vi "test max speed.vi"() -> ()   [LabVIEW 2018]
uses:
  type defs/tet max speed enum.ctl
  <vilib>/Instr/_visa.llb/VISA Configure Serial Port (Instr).vi
panel:
  in  "stop":bool
  out "error IO":errorcluster
  in  "pan tilt stop":bool
  in  "turbo tilt speed":bool
  in  "max tilt speed":bool
  in  "turbo pan speed":bool
  in  "max pan speed":bool
  in  "connect":bool
  in  "VISA resource name":refnum<visa-resource-name>="COM6"
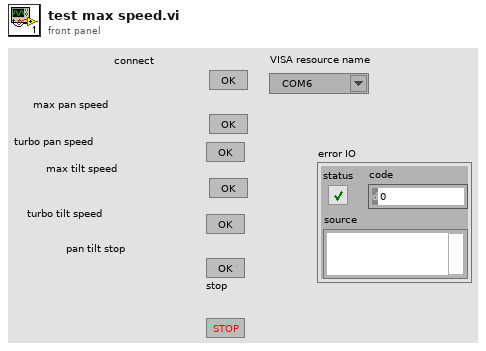
[diagram p1: front panel]
types:
  T1 = typedef "tet max speed enum.ctl" = enum16{"event", "write", "step1", "exit"}
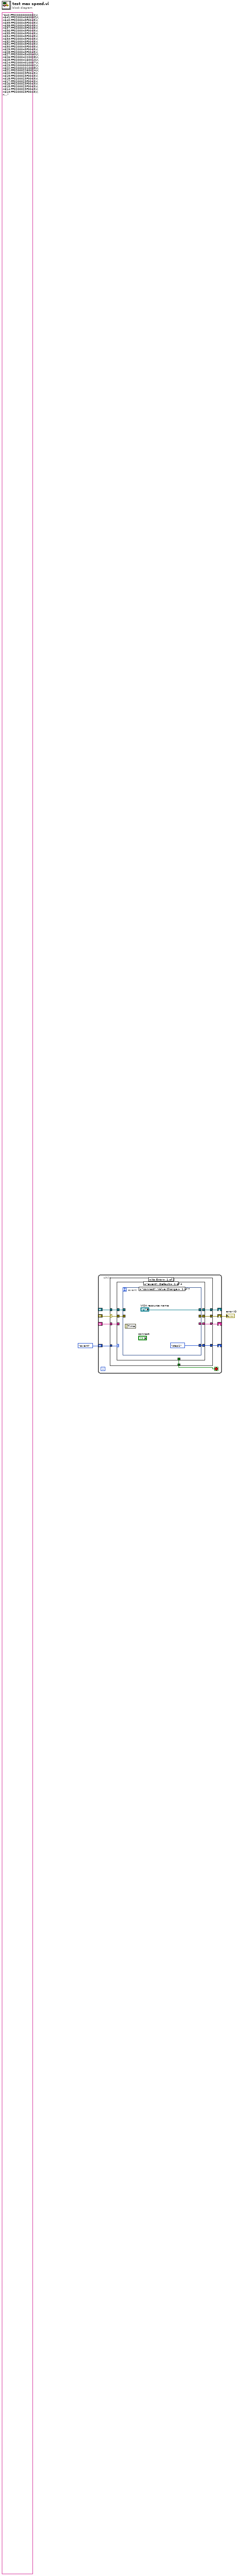
[diagram p0: block diagram]
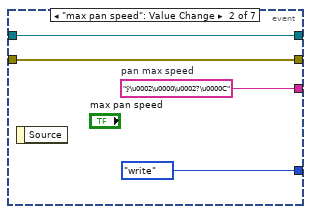
[diagram p2: hidden frame]
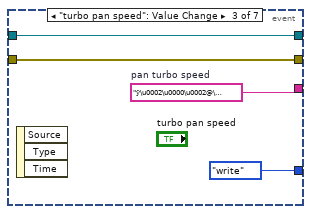
[diagram p3: hidden frame]
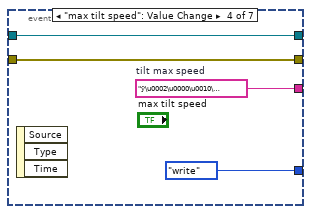
[diagram p4: hidden frame]
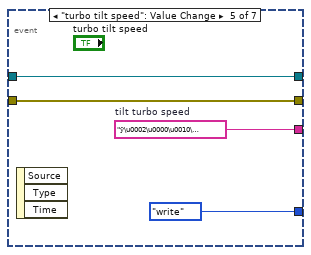
[diagram p5: hidden frame]
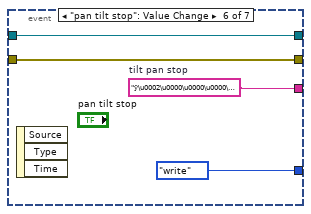
[diagram p6: hidden frame]
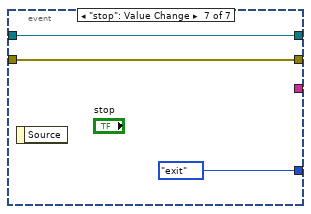
[diagram p7: hidden frame]
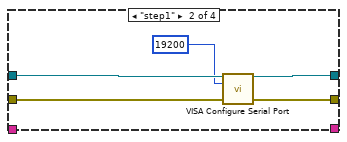
[diagram p8: hidden frame]
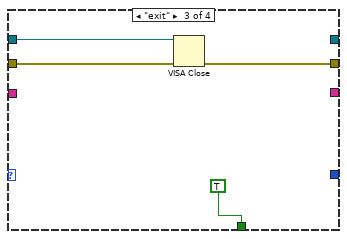
[diagram p9: hidden frame]
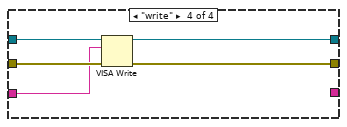
[diagram p10: hidden frame]
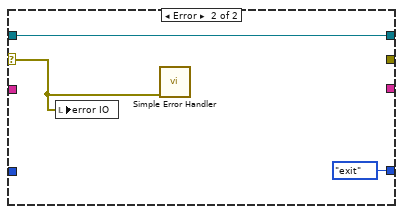
[diagram p11: hidden frame]
diagram:
  (unwired) "642:FF020000000002\r\n641:FF02000406000C\r\n640:FF0200043F0045\r\n639:FF0200043F0045\r\n638:FF0200043F0045\r\n637:FF0200043F0045\r\n636:FF0200043F0045\r\n635:FF0200043F0045\r\n634:FF0200043F0045\r\n633:FF0200043F0045\r\n632:FF0200043F0045\r\n631:FF0200043F0045\r\n630:FF0200043F0045\r\n629:FF0200043F0045\r\n628:FF0200043F0045\r\n627:FF0200043A0040\r\n626:FF020004220028\r\n625:FF02000416001C\r\n624:FF020004010007\r\n623:FF020000000002\r\n622:FF020002010005\r\n621:FF02000226002A\r\n620:FF0200023F0043\r\n619:FF0200023F0043\r\n618:FF0200023F0043\r\n617:FF0200023F0043\r\n616:FF0200023F0043\r\n615:FF0200023F0043\r\n614:FF0200023F0043\r\n613:FF0200023F0043\r\n612:FF0200023F0043\r\n611:FF0200023F0043\r\n610:FF0200023E0042\r\n609:FF02000236003A\r\n608:FF0200021D0021\r\n607:FF020002010005\r\n606:FF0200020E0012\r\n605:FF02000238003C\r\n604:FF0200023F0043\r\n603:FF0200023F0043\r\n602:FF0200023F0043\r\n601:FF0200023F0043\r\n600:FF0200023F0043\r\n599:FF0200023F0043\r\n598:FF0200023F0043\r\n597:FF0200023F0043\r\n596:FF0200023F0043\r\n595:FF02000238003C\r\n594:FF020002240028\r\n593:FF0200021C0020\r\n592:FF020002110015\r\n591:FF020002010005\r\n590:FF0200042A0030\r\n589:FF0200043F0045\r\n588:FF0200043F0045\r\n587:FF0200043F0045\r\n586:FF0200043F0045\r\n585:FF0200043F0045\r\n584:FF0200043F0045\r\n583:FF0200043F0045\r\n582:FF0200043E0044\r\n581:FF0200043F0045\r\n580:FF0200043E0044\r\n579:FF0200043F0045\r\n578:FF0200043F0045\r\n577:FF0200043F0045\r\n576:FF0200043F0045\r\n575:FF0200043F0045\r\n574:FF0200043E0044\r\n573:FF0200043F0045\r\n572:FF0200043F0045\r\n571:FF0200043F0045\r\n570:FF0200043F0045\r\n569:FF0200043F0045\r\n568:FF0200043E0044\r\n567:FF0200043F0045\r\n566:FF0200043F0045\r\n565:FF0200043F0045\r\n564:FF0200043F0045\r\n563:FF0200043E0044\r\n562:FF0200043F0045\r\n561:FF0200043E0044\r\n560:FF020004010007\r\n559:FF020000000002\r\n558:FF020002140018\r\n557:FF0200022E0032\r\n556:FF0200023F0043\r\n555:FF0200023F0043\r\n554:FF0200023F0043\r\n553:FF0200023F0043\r\n552:FF0200023F0043\r\n551:FF0200023F0043\r\n550:FF0200023F0043\r\n549:FF0200023F0043\r\n548:FF0200023F0043\r\n547:FF0200023F0043\r\n546:FF0200023F0043\r\n545:FF0200023F0043\r\n544:FF0200023F0043\r\n543:FF0200023F0043\r\n542:FF0200023F0043\r\n541:FF0200023F0043\r\n540:FF0200023F0043\r\n539:FF0200023F0043\r\n538:FF0200023F0043\r\n537:FF0200023F0043\r\n536:FF0200023F0043\r\n535:FF0200023F0043\r\n534:FF0200023F0043\r\n533:FF0200023F0043\r\n532:FF0200023F0043\r\n531:FF0200023F0043\r\n530:FF0200023F0043\r\n529:FF0200023F0043\r\n528:FF020002340038\r\n527:FF0200022C0030\r\n526:FF020002220026\r\n525:FF020002110015\r\n524:FF020002010005\r\n523:FF0200041E0024\r\n522:FF0200043F0045\r\n521:FF0200043E0044\r\n520:FF0200043F0045\r\n519:FF0200043F0045\r\n518:FF0200043F0045\r\n517:FF0200043F0045\r\n516:FF0200043F0045\r\n515:FF0200043F0045\r\n514:FF0200043F0045\r\n513:FF0200043F0045\r\n512:FF0200043F0045\r\n511:FF0200043E0044\r\n510:FF02000438003E\r\n509:FF02000428002E\r\n508:FF0200040D0013\r\n507:FF020004010007\r\n506:FF020000000002\r\n505:FF02000226002A\r\n504:FF0200023F0043\r\n503:FF0200023F0043\r\n502:FF0200023F0043\r\n501:FF0200023F0043\r\n500:FF0200023F0043\r\n499:FF0200023F0043\r\n498:FF0200023F0043\r\n497:FF0200023F0043\r\n496:FF0200023F0043\r\n495:FF0200023F0043\r\n494:FF0200023F0043\r\n493:FF0200023F0043\r\n492:FF0200023F0043\r\n491:FF0200023F0043\r\n490:FF0200023F0043\r\n489:FF0200023F0043\r\n488:FF0200023F0043\r\n487:FF0200023F0043\r\n486:FF0200023F0043\r\n485:FF0200023F0043\r\n484:FF0200023F0043\r\n483:FF0200023F0043\r\n482:FF0200023F0043\r\n481:FF0200023F0043\r\n480:FF0200023F0043\r\n479:FF0200023F0043\r\n478:FF0200023F0043\r\n477:FF0200023F0043\r\n476:FF0200023F0043\r\n475:FF0200023F0043\r\n474:FF0200023F0043\r\n473:FF0200023F0043\r\n472:FF0200023F0043\r\n471:FF0200023F0043\r\n470:FF0200023F0043\r\n469:FF0200023F0043\r\n468:FF0200023F0043\r\n467:FF0200023F0043\r\n466:FF0200023F0043\r\n465:FF02000229002D\r\n464:FF0200020D0011\r\n463:FF020002010005\r\n462:FF020004100016\r\n461:FF0200043F0045\r\n460:FF0200043F0045\r\n459:FF0200043F0045\r\n458:FF0200043F0045\r\n457:FF0200043F0045\r\n456:FF0200043F0045\r\n455:FF0200043E0044\r\n454:FF0200043F0045\r\n453:FF0200043F0045\r\n452:FF0200043F0045\r\n451:FF0200043F0045\r\n450:FF0200043F0045\r\n449:FF0200043F0045\r\n448:FF0200043F0045\r\n447:FF0200043F0045\r\n446:FF0200043F0045\r\n445:FF0200043E0044\r\n444:FF0200043F0045\r\n443:FF0200043F0045\r\n442:FF0200043E0044\r\n441:FF0200043F0045\r\n440:FF0200043F0045\r\n439:FF0200043F0045\r\n438:FF0200043F0045\r\n437:FF0200043F0045\r\n436:FF0200043F0045\r\n435:FF0200043F0045\r\n434:FF0200043F0045\r\n433:FF0200043E0044\r\n432:FF0200043F0045\r\n431:FF0200043F0045\r\n430:FF02000428002E\r\n429:FF02000419001F\r\n428:FF020004010007\r\n427:FF020000000002\r\n426:FF0200021D0021\r\n425:FF0200022A002E\r\n424:FF02000238003C\r\n423:FF0200023F0043\r\n422:FF0200023F0043\r\n421:FF0200023F0043\r\n420:FF0200023F0043\r\n419:FF0200023F0043\r\n418:FF0200023F0043\r\n417:FF0200023F0043\r\n416:FF0200023F0043\r\n415:FF0200023F0043\r\n414:FF0200023F0043\r\n413:FF0200023F0043\r\n412:FF0200023F0043\r\n411:FF0200023F0043\r\n410:FF0200023F0043\r\n409:FF0200023F0043\r\n408:FF0200023F0043\r\n407:FF0200023F0043\r\n406:FF0200023F0043\r\n405:FF0200023F0043\r\n404:FF0200023F0043\r\n403:FF0200023F0043\r\n402:FF0200023F0043\r\n401:FF0200023F0043\r\n400:FF0200023F0043\r\n399:FF0200023F0043\r\n398:FF0200023F0043\r\n397:FF0200023F0043\r\n396:FF0200023F0043\r\n395:FF0200023F0043\r\n394:FF0200023F0043\r\n393:FF0200023A003E\r\n392:FF020002310035\r\n391:FF0200021C0020\r\n390:FF020002010005\r\n389:FF020000000002\r\n388:FF02000438003E\r\n387:FF0200043F0045\r\n386:FF0200043F0045\r\n385:FF0200043F0045\r\n384:FF0200043F0045\r\n383:FF0200043F0045\r\n382:FF0200043F0045\r\n381:FF0200043F0045\r\n380:FF0200043F0045\r\n379:FF0200043F0045\r\n378:FF0200043E0044\r\n377:FF0200043F0045\r\n376:FF0200043E0044\r\n375:FF0200043F0045\r\n374:FF0200043F0045\r\n373:FF0200043E0044\r\n372:FF0200043F0045\r\n371:FF0200043E0044\r\n370:FF0200043F0045\r\n369:FF02000435003B\r\n368:FF02000424002A\r\n367:FF020004010007\r\n366:FF020000000002\r\n365:FF02000209000D\r\n364:FF02000236003A\r\n363:FF0200023F0043\r\n362:FF0200023F0043\r\n361:FF0200023F0043\r\n360:FF0200023F0043\r\n359:FF0200023F0043\r\n358:FF0200023F0043\r\n357:FF0200023F0043\r\n356:FF0200023F0043\r\n355:FF0200023F0043\r\n354:FF0200023F0043\r\n353:FF0200023F0043\r\n352:FF0200023F0043\r\n351:FF0200023F0043\r\n350:FF0200023F0043\r\n349:FF0200023F0043\r\n348:FF0200023F0043\r\n347:FF0200023F0043\r\n346:FF0200023F0043\r\n345:FF0200023F0043\r\n344:FF0200023F0043\r\n343:FF0200023F0043\r\n342:FF0200023F0043\r\n341:FF0200023F0043\r\n340:FF0200023F0043\r\n339:FF0200023F0043\r\n338:FF0200023F0043\r\n337:FF0200023F0043\r\n336:FF0200023F0043\r\n335:FF0200023F0043\r\n334:FF0200023F0043\r\n333:FF0200023F0043\r\n332:FF0200023F0043\r\n331:FF0200022A002E\r\n330:FF02000219001D\r\n329:FF020002010005\r\n328:FF020000000002\r\n327:FF0200043F0045\r\n326:FF0200043F0045\r\n325:FF0200043F0045\r\n324:FF0200043E0044\r\n323:FF0200043F0045\r\n322:FF0200043F0045\r\n321:FF0200043E0044\r\n320:FF0200043F0045\r\n319:FF0200043E0044\r\n318:FF0200043F0045\r\n317:FF0200043F0045\r\n316:FF0200043F0045\r\n315:FF0200043F0045\r\n314:FF0200043F0045\r\n313:FF0200043F0045\r\n312:FF0200043F0045\r\n311:FF0200043F0045\r\n310:FF0200043F0045\r\n309:FF0200043F0045\r\n308:FF0200043F0045\r\n307:FF0200043E0044\r\n306:FF0200043F0045\r\n305:FF0200043F0045\r\n304:FF0200043F0045\r\n303:FF0200043F0045\r\n302:FF0200043F0045\r\n301:FF0200043F0045\r\n300:FF0200043F0045\r\n299:FF0200043F0045\r\n298:FF0200043F0045\r\n297:FF0200043E0044\r\n296:FF0200043F0045\r\n295:FF0200043F0045\r\n294:FF0200043F0045\r\n293:FF0200043F0045\r\n292:FF0200043F0045\r\n291:FF0200043E0044\r\n290:FF0200043F0045\r\n289:FF0200043F0045\r\n288:FF0200043E0044\r\n287:FF0200043F0045\r\n286:FF020004300036\r\n285:FF020004200026\r\n284:FF020004010007\r\n283:FF020000000002\r\n282:FF020004120018\r\n281:FF02000429002F\r\n280:FF0200042D0033\r\n279:FF020004300036\r\n278:FF020004300036\r\n277:FF020004310037\r\n276:FF020004310037\r\n275:FF020004300036\r\n274:FF020004310037\r\n273:FF020004310037\r\n272:FF020004310037\r\n271:FF020004310037\r\n270:FF020004320038\r\n269:FF020004310037\r\n268:FF0200042E0034\r\n267:FF0200042C0032\r\n266:FF02000428002E\r\n265:FF020004200026\r\n264:FF02000419001F\r\n263:FF0200040E0014\r\n262:FF020004010007\r\n261:FF020000000002\r\n260:FF020002140018\r\n259:FF0200021E0022\r\n258:FF020002200024\r\n257:FF020002200024\r\n256:FF0200021E0022\r\n255:FF0200021D0021\r\n254:FF0200021C0020\r\n253:FF0200021C0020\r\n252:FF0200021A001E\r\n251:FF0200021A001E\r\n250:FF0200021A001E\r\n249:FF02000218001C\r\n248:FF02000218001C\r\n247:FF02000216001A\r\n246:FF020002150019\r\n245:FF020002140018\r\n244:FF020002120016\r\n243:FF020002110015\r\n242:FF0200020D0011\r\n241:FF02000208000C\r\n240:FF020002010005\r\n239:FF020000000002\r\n238:FF020400000006\r\n237:FF020000000002\r\n236:FF020100000003\r\n235:FF020000000002\r\n234:FF020200000004\r\n233:FF020000000002\r\n232:FF020200000004\r\n231:FF020000000002\r\n230:FF020200000004\r\n229:FF020000000002\r\n228:FF020200000004\r\n227:FF020000000002\r\n226:FF020200000004\r\n225:FF020000000002\r\n224:FF020200000004\r\n223:FF020000000002\r\n222:FF020200000004\r\n221:FF020000000002\r\n220:FF020200000004\r\n219:FF020000000002\r\n218:FF020200000004\r\n217:FF020000000002\r\n216:FF020200000004\r\n215:FF020000000002\r\n214:FF02000208000C\r\n213:FF020002100014\r\n212:FF0200020A000E\r\n211:FF02000206000A\r\n210:FF020002010005\r\n209:FF0200040C0012\r\n208:FF0200043F0045\r\n207:FF0200043F0045\r\n206:FF0200043F0045\r\n205:FF0200043F0045\r\n204:FF0200043F0045\r\n203:FF0200043F0045\r\n202:FF0200043D0043\r\n201:FF020004010007\r\n200:FF020000000002\r\n199:FF02000435003B\r\n198:FF0200043F0045\r\n197:FF0200043F0045\r\n196:FF0200043E0044\r\n195:FF0200043F0045\r\n194:FF0200043F0045\r\n193:FF0200043F0045\r\n192:FF0200043F0045\r\n191:FF0200043F0045\r\n190:FF0200043F0045\r\n189:FF0200043F0045\r\n188:FF0200043F0045\r\n187:FF0200042A0030\r\n186:FF020004010007\r\n185:FF020000000002\r\n184:FF0200020A000E\r\n183:FF02000238003C\r\n182:FF0200023F0043\r\n181:FF0200023F0043\r\n180:FF0200023F0043\r\n179:FF0200023F0043\r\n178:FF0200023F0043\r\n177:FF0200023F0043\r\n176:FF0200023F0043\r\n175:FF0200023F0043\r\n174:FF0200023F0043\r\n173:FF0200023F0043\r\n172:FF0200023F0043\r\n171:FF0200023C0040\r\n170:FF0200022D0031\r\n169:FF020002010005\r\n168:FF020000000002\r\n167:FF020002120016\r\n166:FF0200023F0043\r\n165:FF0200023F0043\r\n164:FF0200023F0043\r\n163:FF0200023F0043\r\n162:FF0200023F0043\r\n161:FF0200023F0043\r\n160:FF0200023F0043\r\n159:FF0200023F0043\r\n158:FF0200023F0043\r\n157:FF0200023F0043\r\n156:FF0200023F0043\r\n155:FF0200023F0043\r\n154:FF0200023F0043\r\n153:FF0200023F0043\r\n152:FF0200023F0043\r\n151:FF0200023F0043\r\n150:FF0200023F0043\r\n149:FF0200023F0043\r\n148:FF0200023F0043\r\n147:FF02000236003A\r\n146:FF020002300034\r\n145:FF0200021D0021\r\n144:FF020002010005\r\n143:FF020004100016\r\n142:FF0200043F0045\r\n141:FF0200043F0045\r\n140:FF0200043F0045\r\n139:FF0200043F0045\r\n138:FF0200043F0045\r\n137:FF0200043F0045\r\n136:FF0200043E0044\r\n135:FF0200043F0045\r\n134:FF0200043F0045\r\n133:FF0200043F0045\r\n132:FF0200043F0045\r\n131:FF0200043F0045\r\n130:FF02000414001A\r\n129:FF020004010007\r\n128:FF02000218001C\r\n127:FF020002350039\r\n126:FF0200023F0043\r\n125:FF0200023F0043\r\n124:FF0200023F0043\r\n123:FF0200023F0043\r\n122:FF02000236003A\r\n121:FF020002210025\r\n120:FF020002010005\r\n119:FF02000206000A\r\n118:FF02000218001C\r\n117:FF0200022A002E\r\n116:FF0200023F0043\r\n115:FF0200023F0043\r\n114:FF0200023F0043\r\n113:FF0200023F0043\r\n112:FF0200023F0043\r\n111:FF0200023F0043\r\n110:FF0200023F0043\r\n109:FF0200023F0043\r\n108:FF0200023F0043\r\n107:FF0200023F0043\r\n106:FF0200023F0043\r\n105:FF0200023F0043\r\n104:FF02000238003C\r\n103:FF020002350039\r\n102:FF020002220026\r\n101:FF020002010005\r\n100:FF020000000002\r\n99:FF02000424002A\r\n98:FF0200043E0044\r\n97:FF0200043F0045\r\n96:FF0200043E0044\r\n95:FF0200043F0045\r\n94:FF0200043F0045\r\n93:FF0200043F0045\r\n92:FF0200043F0045\r\n91:FF0200043E0044\r\n90:FF0200043F0045\r\n89:FF0200043F0045\r\n88:FF0200043F0045\r\n87:FF0200043F0045\r\n86:FF0200043F0045\r\n85:FF020004310037\r\n84:FF020004010007\r\n83:FF02000414001A\r\n82:FF0200042E0034\r\n81:FF0200043F0045\r\n80:FF0200043E0044\r\n79:FF0200043F0045\r\n78:FF0200043F0045\r\n77:FF0200043F0045\r\n76:FF0200043F0045\r\n75:FF0200043F0045\r\n74:FF0200043F0045\r\n73:FF0200043F0045\r\n72:FF0200043F0045\r\n71:FF0200043F0045\r\n70:FF0200043F0045\r\n69:FF0200043F0045\r\n68:FF0200043F0045\r\n67:FF0200043F0045\r\n66:FF0200043E0044\r\n65:FF0200043F0045\r\n64:FF0200043E0044\r\n63:FF0200043F0045\r\n62:FF0200043F0045\r\n61:FF0200043F0045\r\n60:FF0200043F0045\r\n59:FF0200043F0045\r\n58:FF0200043F0045\r\n57:FF0200043F0045\r\n56:FF0200043F0045\r\n55:FF0200043F0045\r\n54:FF0200043F0045\r\n53:FF02000434003A\r\n52:FF02000429002F\r\n51:FF020004120018\r\n50:FF020004010007\r\n49:FF020000000002\r\n48:FF020200000004\r\n47:FF020000000002\r\n46:FF020200000004\r\n45:FF010000000001\r\n44:FF010200000003\r\n43:FF010000000001\r\n42:FF010200000003\r\n41:FF010000000001\r\n40:FF010200000003\r\n39:FF010000000001\r\n38:FF010200000003\r\n37:FF010000000001\r\n36:FF010200000003\r\n35:FF010000000001\r\n34:FF010200000003\r\n33:FF010000000001\r\n32:FF010200000003\r\n31:FF0100020A000D\r\n30:FF010002360039\r\n29:FF0100023F0042\r\n28:FF0100023F0042\r\n27:FF0100023F0042\r\n26:FF0100023F0042\r\n25:FF0100023E0041\r\n24:FF0100022C002F\r\n23:FF0100021C001F\r\n22:FF010002010004\r\n21:FF010000000001\r\n20:FF01000415001A\r\n19:FF0100042C0031\r\n18:FF0100043F0044\r\n17:FF0100043F0044\r\n16:FF0100043F0044\r\n15:FF0100043F0044\r\n14:FF0100043F0044\r\n13:FF0100043E0043\r\n12:FF0100043F0044\r\n11:FF01000438003D\r\n10:FF01000426002B\r\n9:FF01000416001B\r\n8:FF010004010006\r\n7:FF010000000001\r\n6:FF010200000003\r\n5:FF010000000001\r\n4:FF010200000003\r\n3:FF010000000001\r\n2:FF010200000003\r\n1:FF010000000001\r\n0:FF010200000003\r\n" ("keypad cmd")
  n1 = while {
    shift-right: [w7] -> _
    shift-left: tet_max_speed_enum."event" -> [w11]
    shift-right: [w9] -> _
    shift-left: _ -> [w8]
    shift-right: [w6] -> w1
    shift-left: _ -> [w3]
    shift-right: [w5] -> _
    shift-left: _ -> [w4]
    stop <- w10 stop-if-true
    n2 = case shown="No Error" w3 {
      selector: w3 -> [w12 w66]
      tunnel: w11 -> [w20 _]
      tunnel: [w19 _] -> w10
      tunnel: [w18 w67] -> w9
      tunnel: w8 -> [w17 w67]
      tunnel: [w16 tet_max_speed_enum."exit"] -> w7
      tunnel: [w15 _] -> w6
      tunnel: [w14 _] -> w5
      tunnel: w4 -> [w13 _]
      frame No Error {
        n3 = case shown="\"event\", Default" w20 {
          tunnel: [_ _ TRUE _] -> w19
          tunnel: [w25 w56 _ w64] -> w18
          tunnel: w17 -> [w26 w55 w59 w65]
          tunnel: [w24 _ _ _] -> w16
          tunnel: [w22 w53 w58 w62] -> w15
          tunnel: w12 -> [w21 w52 w57 w63]
          tunnel: [w23 _ _ _] -> w14
          tunnel: w13 -> [_ _ _ w61]
          frame "event", Default {
            n4 = event shown="[0] \"connect\": Value Change" {
              selector: _ -> [_ _ _ _ _ _ _]
              dyn-events: _ -> [_ _ _ _ _ _ _]
              timeout: _ -> [_ _ _ _ _ _ _]
              tunnel: w26 -> [_ w30 w36 w38 w42 w48 w51]
              tunnel: ["VISA resource name" w30 w36 w38 w42 w48 w51] -> w25
              tunnel: [tet_max_speed_enum."step1" tet_max_speed_enum."write" tet_max_speed_enum."write" tet_max_speed_enum."write" tet_max_speed_enum."write" tet_max_speed_enum."write" tet_max_speed_enum."exit"] -> w24
              tunnel: [_ w32 w34 w40 w44 w46 _] -> w23
              tunnel: [_ w29 w35 w39 w41 w47 w50] -> w22
              tunnel: w21 -> [_ w29 w35 w39 w41 w47 w50]
              event "connect": Value Change {
                n5 = event-data() -> ()  [unwired: 1 in, 1 out]
              }
              event "max pan speed": Value Change {
                w32 = "ÿ\u0002\u0000\u0002?\u0000C"  # pan max speed
                n6 = event-data() -> ()  [unwired: 1 in, 1 out]
              }
              event "turbo pan speed": Value Change {
                w34 = "ÿ\u0002\u0000\u0002@\u0000D"  # pan turbo speed
                n7 = event-data() -> ()  [unwired: 1 in, 3 out]
              }
              event "max tilt speed": Value Change {
                w40 = "ÿ\u0002\u0000\u0010\u0000?Q"  # tilt max speed
                n8 = event-data() -> ()  [unwired: 1 in, 3 out]
              }
              event "turbo tilt speed": Value Change {
                w44 = "ÿ\u0002\u0000\u0010\u0000@R"  # tilt turbo speed
                n9 = event-data() -> ()  [unwired: 1 in, 3 out]
              }
              event "pan tilt stop": Value Change {
                w46 = "ÿ\u0002\u0000\u0000\u0000\u0000\u0002"  # tilt pan stop
                n10 = event-data() -> ()  [unwired: 1 in, 3 out]
              }
              event "stop": Value Change {
                n11 = event-data() -> ()  [unwired: 1 in, 1 out]
              }
            }
          }
          frame "step1" {
            n12 = call-poly "VISA Configure Serial Port"("VISA resource name"=w55, "baud rate (9600)"=u32 19200, "error in (no error)"=w52) -> ("VISA resource name out"=w56:refnum<visa-resource-name>, "error out"=w53:errorcluster)  [unwired: 11 in]
          }
          frame "exit" {
            n13 = VISA Close(VISA resource name=w59, error in (no error)=w57) -> (error out=w58:errorcluster)
          }
          frame "write" {
            n14 = VISA Write(VISA resource name=w65, write buffer=w61, error in (no error)=w63) -> (VISA resource name out=w64:refnum<visa-resource-name>, error out=w62:errorcluster)  [unwired: 1 out]
          }
        }
      }
      frame Error {
        n15 = local write "error IO"(w66) -> ()
        n16 = call <vilib>:"Simple Error Handler.vi"("error in (no error)"=w66) -> ()  [unwired: 4 in, 5 out]
      }
    }
  }
  "error IO" <- w1
